vi "Flush Data to Log File.vi"(8 "error in (no error)":T1 caption="entrée d'erreur (pas d'erreur)", 10 "File d'attente de données":refnum<queue>, 11 "Configuration de l'enregistrement":T2) -> (0 "error out":T1 caption="sortie d'erreur")   [LabVIEW 2020, in "Logging.lvlib"]
doc: "Retirer de la file d'attente toutes les données en attente et les écrire dans le fichier journal. Fermer la référence de fichier TDMS."
uses:
  Logging.lvlib
  Logging Configuration.ctl
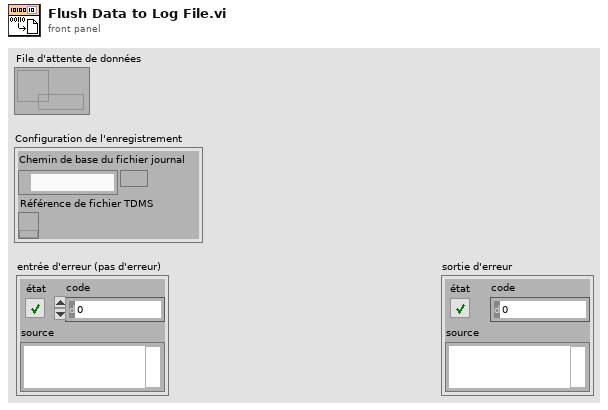
[diagram p1: front panel]
types:
  T1 = cluster{"état":bool, "code":i32, "source":string}
  T2 = typedef "Logging.lvlib/Logging Configuration.ctl" = cluster{"Chemin de base du fichier journal":path, "Référence de fichier TDMS":refnum<k34>}
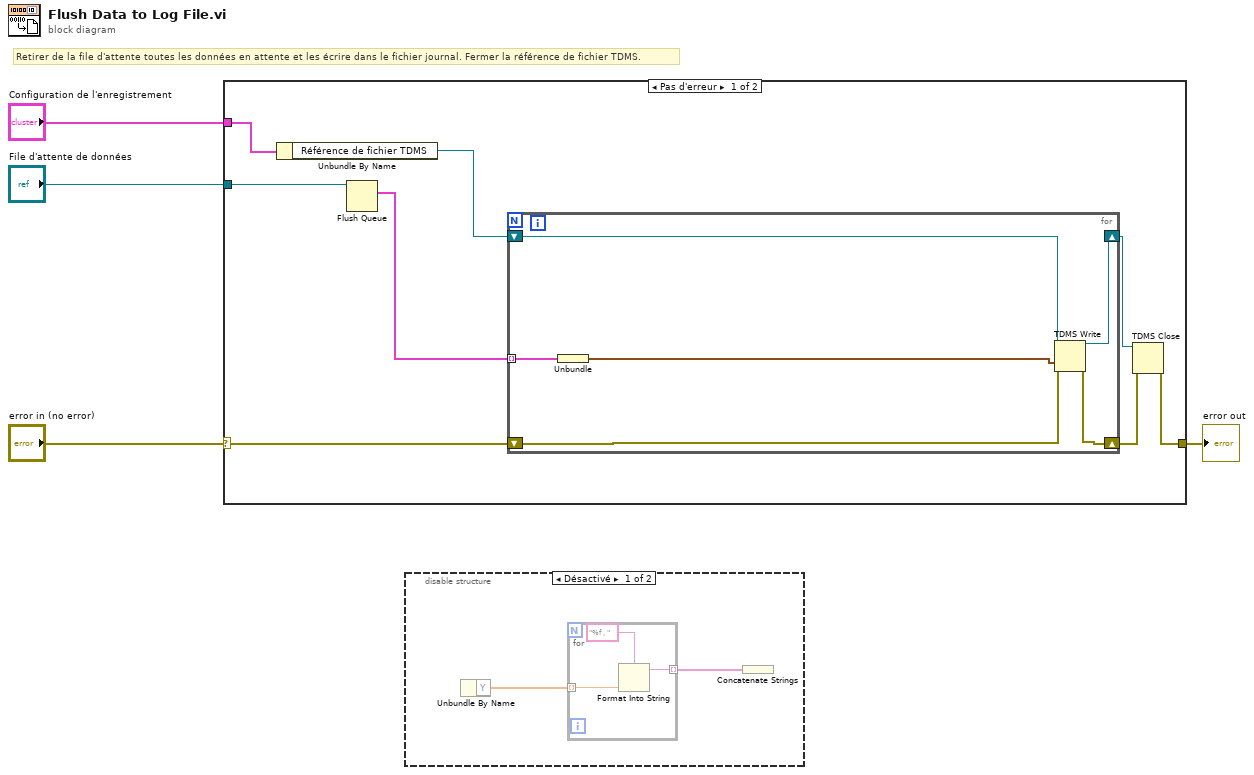
[diagram p0: block diagram]
diagram:
  # "Retirer de la file d'attente toutes les données en attente et les écrire dans le fichier journal. Fermer la référence de fichier TDMS."
  n1 = case shown="Pas d'erreur" "error in (no error)" {
    selector: "error in (no error)" -> [w5 w19]
    tunnel: "File d'attente de données" -> [w8 _]
    tunnel: "Configuration de l'enregistrement" -> [w7 _]
    tunnel: [w6 w19] -> w2
    frame No Error {
      n2 = Unbundle By Name(w7) -> ("Référence de fichier TDMS"=w9:refnum<k34>)
      n3 = Flush Queue(queue=w8) -> (remaining elements=w12:cluster{"Array":waveform(dbl)[]}[])  [unwired: 1 in, 2 out]
      n4 = for {
        shift-right: [w16] -> w10
        shift-left: w9 -> [w17]
        shift-right: [w18] -> w11
        shift-left: w5 -> [w15]
        tunnel: w12 -> [w13] mode=indexing
        n5 = Unbundle(w13) -> ("Array"=w14:waveform(dbl)[])
        n6 = TDMS Write(0:w17, 9:w14, 11:w15) -> (4:w16:refnum<k34>, 15:w18:errorcluster)  [unwired: 3 in, 2 out]
      }
      n7 = TDMS Close(8:w11, 11:w10) -> (0:w6:errorcluster)  [unwired: 1 out]
    }
    frame Error {
    }
  }
  "error out" <- w2
  n8 = disable-structure shown="Désactivé" {
    frame Disabled {
      n9 = Unbundle By Name() -> ("Y"=w20:dbl[])  [unwired: 1 in]
      n10 = for {
        tunnel: w20 -> [w24] mode=indexing
        tunnel: [w23] -> w21 mode=indexing
        n11 = Format Into String(format string="%f , ", w24) -> (resulting string=w23:string)  [unwired: 2 in, 1 out]
      }
      n12 = Concatenate Strings(w21) -> ()  [unwired: 1 out]
    }
    frame Enabled {
    }
  }
